vi "ARREGLOS DIMENSIONALES.vi"(6 "CANTIDAD":i64[](array[numeric]), 9 "MONEDA":string[](array[string]), 10 "PRODUCTO":string[](array[string]), 11 "COSTO":i64[](array[numeric])) -> (2 "Array":string[][](array[string]))   [LabVIEW 2019, in "DATA_UI_CAFÉ_MEX_ESP.lvlib" / "UI_CAFÉ_MEX_ESP.lvclass"]
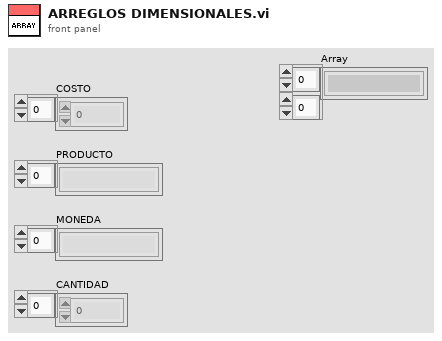
[diagram p1: front panel]
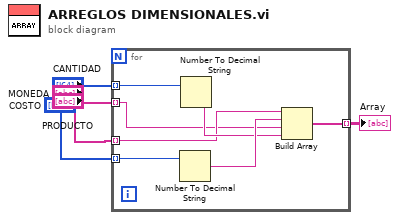
[diagram p0: block diagram]
diagram:
  n1 = for {
    tunnel: [w10] -> w1 mode=indexing
    tunnel: "CANTIDAD" -> [w9] mode=indexing
    tunnel: "COSTO" -> [w8] mode=indexing
    tunnel: "MONEDA" -> [w6] mode=indexing
    tunnel: "PRODUCTO" -> [w7] mode=indexing
    n2 = Number To Decimal String(number=w8) -> (decimal integer string=w12:string)  [unwired: 1 in]
    n3 = Number To Decimal String(number=w9) -> (decimal integer string=w11:string)  [unwired: 1 in]
    n4 = Build Array(w7, w12, w6, w11) -> (w10:string[])
  }
  "Array" <- w1
